vi "Send Message.vi"(0 "ICanCommunicate In":refnum<class "Process.lvclass">, 7 "Message":T1, 11 "Error In":errorcluster) -> (4 "ICanCommunicate Out":refnum<class "Process.lvclass">, 15 "Error Out":errorcluster)   [LabVIEW 2023, in "Process.lvclass"]
uses:
  Process.lvclass
  Interfaces/ICanCommunicate/Message.ctl
  Interfaces/ICanCommunicate/ICanCommunicate.lvclass
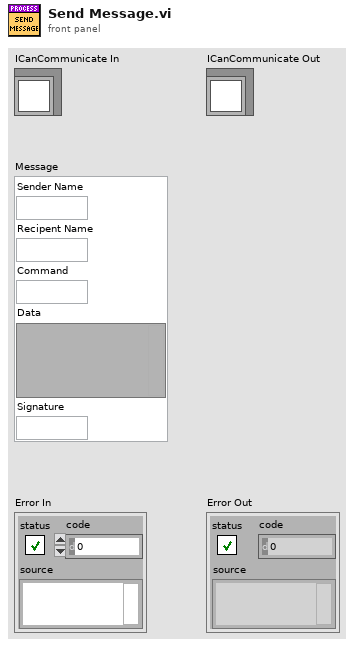
[diagram p1: front panel]
types:
  T1 = typedef "ICanCommunicate.lvclass/Message.ctl" = cluster{"Sender Name":string, "Recipent Name":string, "Command":string, "Data":variant, "Signature":string}
  T2 = typedef "ICanCommunicate.lvclass/ToProcessQueue.ctl" = refnum<queue>
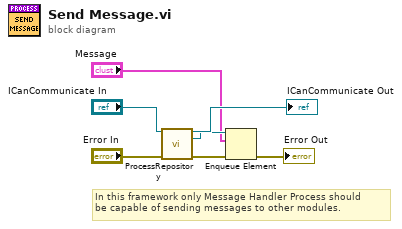
[diagram p0: block diagram]
diagram:
  # "In this framework only Message Handler Process should\nbe capable of sending messages to other modules."
  n1 = call-dynamic "ProcessRepository.vi"("Process In"="ICanCommunicate In", "Error In"="Error In") -> ("Process Out"=→"ICanCommunicate Out":refnum<class "Process.lvclass">, "ToProcessQueue"=w5:T2, "Error Out"=w4:errorcluster)  [unwired: 7 in, 4 out]
  n2 = Enqueue Element(queue=w5, element="Message", error in (no error)=w4) -> (error out=→"Error Out":errorcluster)  [unwired: 1 in, 2 out]
